vi "校准基准_control switch.vi"(8 "error in (no error)":errorcluster, 9 "COM":i32, 11 "A":i32) -> (0 "error out":errorcluster)   [LabVIEW 2011]
uses:
  network_Global/Global.vi
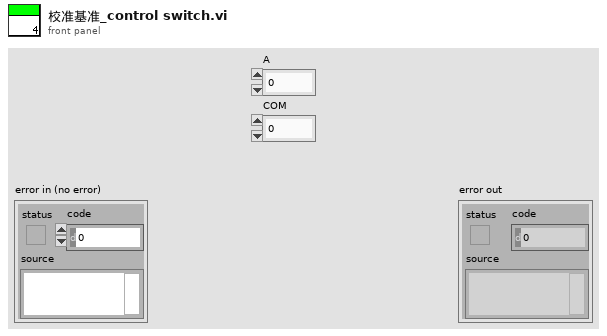
[diagram p1: front panel]
types:
  T1 = typedef "通道.ctl" = cluster{"用户名":string, "RF进口":string, "RF出口":string, "CLK进口":string, "CLK出口":string, "FCLK进口":string, "FCLK出口":string, "时间":u16}
  T2 = cluster{"用户名":string, "RF进口":string, "RF出口":string, "CLK进口":string, "CLK出口":string, "FCLK进口":string, "FCLK出口":string, "时间":u16}
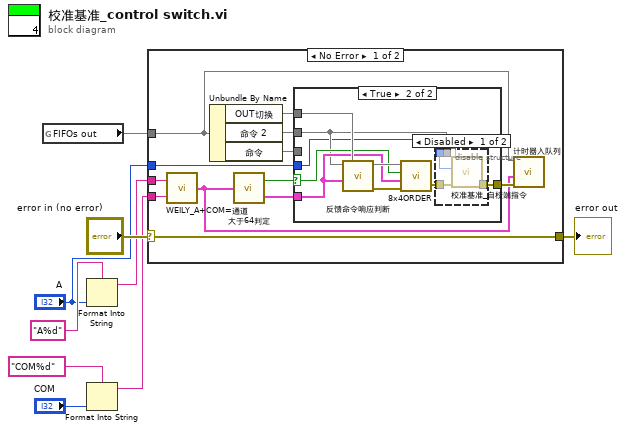
[diagram p0: block diagram]
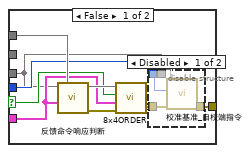
[diagram p2: hidden frame]
diagram:
  n1 = global read "Global.vi" "FIFOs out"() -> (w7)
  n2 = Format Into String(format string="A%d", "A") -> (resulting string=w3:string)  [unwired: 2 in, 1 out]
  n3 = Format Into String(format string="COM%d", "COM") -> (resulting string=w2:string)  [unwired: 2 in, 1 out]
  n4 = case shown="No Error" "error in (no error)" {
    selector: "error in (no error)" -> [w21 w48]
    tunnel: [w21 w48] -> w8
    tunnel: w7 -> [w15 _]
    tunnel: w3 -> [w12 _]
    tunnel: w2 -> [w11 _]
    tunnel: "A" -> [w10 _]
    frame No Error {
      n5 = call "WEILY_A+COM=通道.vi"("RF出口"=w11, "RF进口"=w12) -> ("通道"=w13:T1)
      n6 = Unbundle By Name(w15) -> ("OUT切换"=w18, "命令 2"=w17, "命令"=w16)
      n7 = call "大于64判定.vi"("通道"=w13) -> (">64"=w20:bool, "通道(出)"=w19:T2)
      n8 = case shown="True" w20 {
        selector: w20 -> [w27 w40]
        tunnel: [w24 w37] -> w14
        tunnel: w16 -> [w22 _]
        tunnel: w19 -> [w26 w39]
        tunnel: w17 -> [_ w36]
        tunnel: w18 -> [w28 w41]
        tunnel: w10 -> [w23 w35]
        frame False {
          n9 = call "反馈命令响应判断.vi"("通道"=w26, "命令"=w22) -> ("error out"=w29:errorcluster)  [unwired: 5 in]
          n10 = call "8x4ORDER.vi"("error in"=w29, "通道"=w26, ">64"=w27, "OUT切换"=w28) -> ("error out"=w25:errorcluster)  [unwired: 1 out]
          n11 = disable-structure shown="Disabled" {
            disable-tunnel: w25 -> [w33 w34]
            disable-tunnel: [w32 w34] -> w24
            disable-tunnel: w23 -> [w31 _]
            disable-tunnel: w22 -> [w30 _]
            frame Disabled {
              n12 = call "校准基准_自校端指令.vi"("error in (no error)"=w33, "进口"=w31, "命令"=w30) -> ("error out"=w32:errorcluster)  [unwired: 8 in]
            }
            frame Enabled {
            }
          }
        }
        frame True {
          n13 = call "反馈命令响应判断.vi"("通道"=w39, "命令"=w36) -> ("error out"=w42:errorcluster)  [unwired: 5 in]
          n14 = call "8x4ORDER.vi"("error in"=w42, "通道"=w39, ">64"=w40, "OUT切换"=w41) -> ("error out"=w38:errorcluster)  [unwired: 1 out]
          n15 = disable-structure shown="Disabled" {
            disable-tunnel: w38 -> [w46 w47]
            disable-tunnel: [w45 w47] -> w37
            disable-tunnel: w36 -> [w44 _]
            disable-tunnel: w35 -> [w43 _]
            frame Disabled {
              n16 = call "校准基准_自校端指令.vi"("error in (no error)"=w46, "进口"=w43, "命令"=w44) -> ("error out"=w45:errorcluster)  [unwired: 8 in]
            }
            frame Enabled {
            }
          }
        }
      }
      n17 = call "计时器入队列.vi"("error in"=w14, "通道"=w13, "FIFOs in"=w15) -> ()  [unwired: 4 in, 1 out]
    }
    frame Error {
    }
  }
  "error out" <- w8
